vi "set-wnum.vi"(10 "wnum":dbl=2284.249 format="%#_13g") -> (0 "error out":errorcluster)   [LabVIEW 2014]
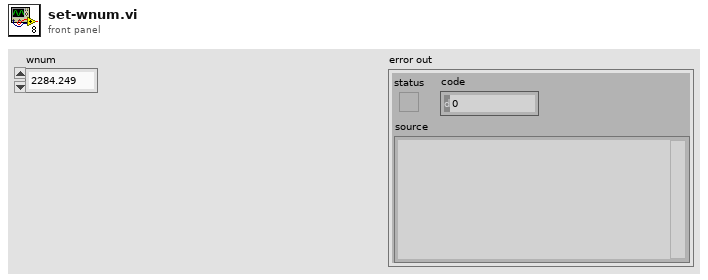
[diagram p1: front panel]
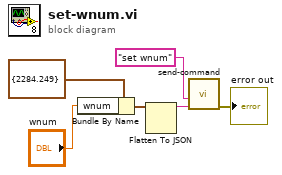
[diagram p0: block diagram]
diagram:
  n1 = Bundle By Name(cluster=cluster{"wnum":dbl} {"wnum"=2284.249}, "wnum"="wnum") -> (w1:cluster{"wnum":dbl})
  n2 = Flatten To JSON(anything=w1) -> (JSON string=w5:string)  [unwired: 2 in, 1 out]
  n3 = call "send-command.vi"("parameters"=w5, "command"="set wnum") -> ("error out"=→"error out":errorcluster)  [unwired: 8 in, 1 out]
